vi "ICS425.vi"(0 "VISA resource name":refnum<visa-resource-name>="SETRA", 11 "Error In":errorcluster) -> (15 "Error Out":errorcluster)   [LabVIEW 2020]
panel:
  out "concatenated string":string
  in  "Commad":string
  out "Read Buffer":string
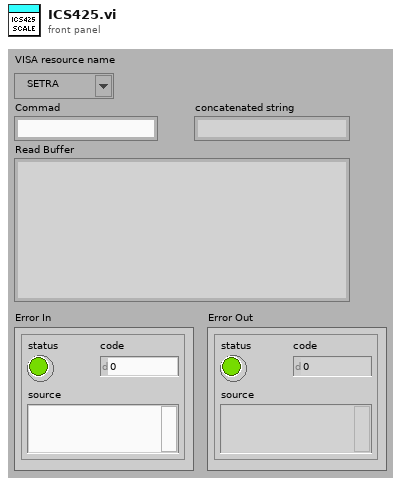
[diagram p1: front panel]
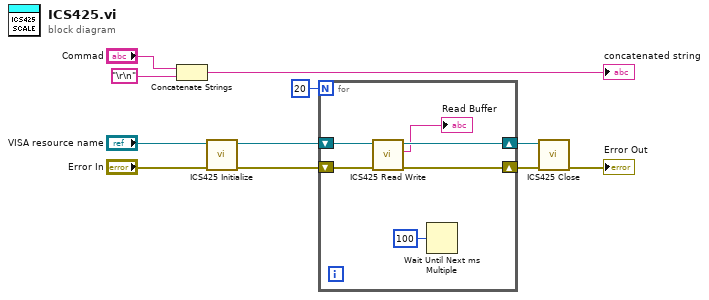
[diagram p0: block diagram]
diagram:
  n1 = Concatenate Strings("Commad", "\r\n") -> (→"concatenated string":string)
  n2 = call "ICS425 Initialize.vi"("Error In"="Error In", "VISA Refnum in"="VISA resource name") -> ("Error Out"=w2:errorcluster, "VISA Refnum out"=w9:refnum<visa-resource-name>)  [unwired: 8 in]
  n3 = for {
    N: 20 -> [_]
    shift-right: [w16] -> w8
    shift-left: w9 -> [w17]
    shift-right: [w15] -> w7
    shift-left: w2 -> [w14]
    n4 = call "ICS425 Read Write.vi"("Error In"=w14, "VISA (Input)"=w17) -> ("Error Out"=w15:errorcluster, "read buffer"=→"Read Buffer":string, "VISA Refnum (Output)"=w16:refnum<visa-resource-name>)  [unwired: 7 in]
    n5 = Wait Until Next ms Multiple(millisecond multiple=u32 100) -> ()  [unwired: 1 out]
  }
  n6 = call "ICS425 Close.vi"("Error In"=w7, "VISA Refnum in"=w8) -> ("Error Out"=→"Error Out":errorcluster)  [unwired: 9 in]
